vi "svfa_Tone Estimation (complex).vi"(8 "FFT size":i32, 9 "window size":i32, 10 "window":T1(ring), 11 "three fingers":cluster{"f0":dbl, "df":dbl, "spectrum":cdb[]}={"f0"=0.0, "df"=1.0, "spectrum"=[]} {"spectrum" format="%.2f"; "df" format="%.2f"; "f0" format="%.5f"}) -> (3 "single tone info.":T2 {"phase [degree]" format="%.2f"; "amplitude" format="%_6f"; "frequency" format="%_16e"})   [LabVIEW 2017]
doc: "This VI takes the three domainent FFT bins to apply the Newton-Raphson's root finding algorithm to determine the exact frequency, phase and amplitude.\nThe input is not necessary \"three fingers\", it could be two, four, or more."
uses:
  <vilib>/addons/_NISVFA/_Spectrum Processing/subVIs/svfa_Tone Estimation Subroutine G(f) (complex).vi
  <vilib>/addons/_NISVFA/_Spectrum Processing/subVIs/svfa_Window Frequency Response.vi
  <vilib>/addons/_NISVFA/_Spectrum Processing/subVIs/svfa_Window Frequency Response (double array).vi
  <vilib>/Analysis/baseanly.llb/Dot Product.vi
  <vilib>/Analysis/baseanly.llb/Complex Dot Product.vi
  <vilib>/addons/_NISVFA/_Spectrum Processing/subVIs/svfa_Rect Window Frequency Response.vi
  <vilib>/addons/_NISVFA/_Spectrum Processing/subVIs/svfa_Tone Estimation Subroutine G(f) (first derivative) (complex).vi
  <vilib>/addons/_NISVFA/_Spectrum Processing/subVIs/svfa_Cosine Window Coefficients.vi
  <vilib>/addons/_NISVFA/_Spectrum Processing/subVIs/svfa_Initial Guess for Tone Estimation (complex).vi
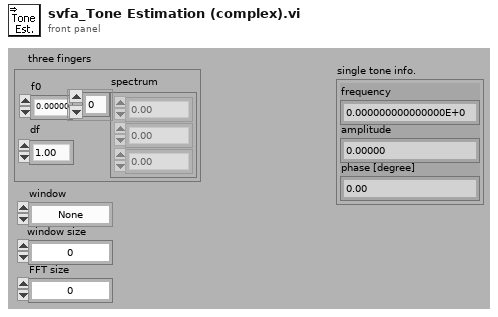
[diagram p1: front panel]
types:
  T1 = enum16{"None ", "Hanning", "Hamming", "Blackman-Harris", "Exact Blackman", "Blackman", "Flat Top", "4 Term B-Harris ", "7 Term B-Harris", "Low Sidelobe"}
  T2 = cluster{"frequency":dbl, "amplitude":dbl, "phase [degree]":dbl}
  T3 = cluster{"initial guess":dbl, "Amplitude":dbl, "initial guess":dbl}
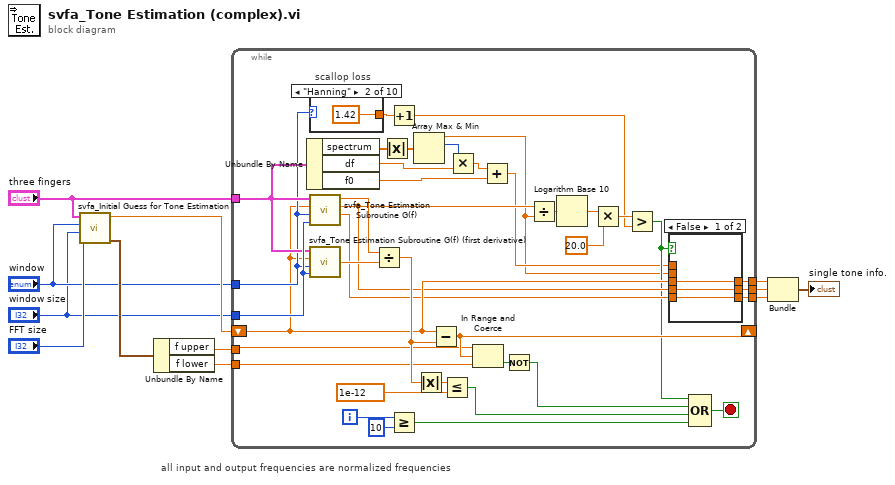
[diagram p0: block diagram]
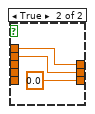
[diagram p2: hidden frame]
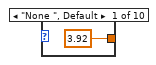
[diagram p3: hidden frame]
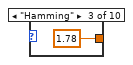
[diagram p4: hidden frame]
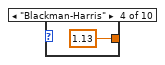
[diagram p5: hidden frame]
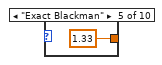
[diagram p6: hidden frame]
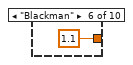
[diagram p7: hidden frame]
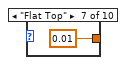
[diagram p8: hidden frame]
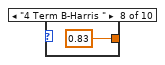
[diagram p9: hidden frame]
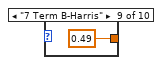
[diagram p10: hidden frame]
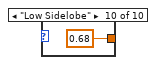
[diagram p11: hidden frame]
diagram:
  # "all input and output frequencies are normalized frequencies"
  n1 = call-poly <vilib>:"svfa_Initial Guess for Tone Estimation.vi"("FFT size"="FFT size", "window size"="window size", "window"="window", "three fingers"="three fingers") -> ("range"=w5:cluster{"f upper":dbl, "f lower":dbl}, "initial guess"=w4:dbl)  [unwired: 6 in]
  n2 = Unbundle By Name(w5) -> ("f upper"=w9:dbl, "f lower"=w8:dbl)
  n3 = while {
    tunnel: "three fingers" -> [w36]
    tunnel: w8 -> [w38]
    tunnel: "window size" -> [w37]
    tunnel: "window" -> [w33]
    tunnel: w9 -> [w39]
    tunnel: [w25] -> w11
    tunnel: [w26] -> w10
    tunnel: [w27] -> w7
    shift-left: w4 -> [w30]
    shift-right: [w41] -> _
    i -> [w45]
    stop <- w47 stop-if-true
    # "scallop loss"
    n4 = Unbundle By Name(w36) -> ("spectrum"=w35:cdb[], "df"=w21:dbl, "f0"=w20:dbl)
    n5 = case shown="\"Hanning\"" w33 {
      tunnel: [3.92 ("y") 1.42 ("y") 1.78 ("y") 1.13 ("y") 1.33 ("y") 1.1 ("y") 0.01 ("y") 0.83 ("y") 0.49 ("y") 0.68 ("y")] -> w31
      frame "None ", Default {
      }
      frame "Hanning" {
      }
      frame "Hamming" {
      }
      frame "Blackman-Harris" {
      }
      frame "Exact Blackman" {
      }
      frame "Blackman" {
      }
      frame "Flat Top" {
      }
      frame "4 Term B-Harris " {
      }
      frame "7 Term B-Harris" {
      }
      frame "Low Sidelobe" {
      }
    }
    n6 = call-poly <vilib>:"svfa_Tone Estimation Subroutine G(f).vi"("N (window length)"=w37, "window"=w33, "frequency"=w30, "three fingers"=w36) -> ("phase [degree]"=w28:dbl, "Amplitude"=w29:dbl, "G(f)"=w42:dbl)  [unwired: 1 in]
    n7 = call-poly <vilib>:"svfa_Tone Estimation Subroutine G(f) (first derivative).vi"("N (window length)"=w37, "window"=w33, "frequency"=w30, "three fingers"=w36) -> ("G'(f)"=w51:dbl)
    n8 = Divide(x=w42, y=w51) -> (x/y=w46:dbl)
    n9 = Absolute Value(x=w35) -> (abs(x)=w34:dbl[])
    n10 = Increment(x=w31) -> (x+1=w13:dbl)
    n11 = Greater Or Equal?(x=w45, y=10) -> (x >= y?=w48:bool)
    n12 = Array Max & Min(array=w34) -> (max value=w17:dbl, max index (indices)=w22:i32)  [unwired: 2 out]
    n13 = Absolute Value(x=w46) -> (abs(x)=w49:dbl)
    n14 = Subtract(x=w30, y=w46) -> (x-y=w41:dbl)
    n15 = Less Or Equal?(x=w49, y=1e-12) -> (x <= y?=w43:bool)
    n16 = Multiply(x=w22, y=w21) -> (x*y=w19:dbl)
    n17 = In Range and Coerce(upper limit=w39, x=w41, lower limit=w38) -> (In Range?=w40:bool)  [unwired: 1 out]
    n18 = Add(x=w19, y=w20) -> (x+y=w18:dbl)
    n19 = Not(x=w40) -> (.not. x?=w24:bool)
    n20 = Divide(x=w29, y=w17) -> (x/y=w32:dbl)
    n21 = Logarithm Base 10(1:w32) -> (0:w16:dbl)
    n22 = Multiply(x=w16, y=20.0) -> (x*y=w15:dbl)
    n23 = Greater?(x=w15, y=w13) -> (0:w23:bool)
    n24 = case shown="False" w23 {
      tunnel: w30 -> [w54 _]
      tunnel: w29 -> [w53 _]
      tunnel: w28 -> [w52 _]
      tunnel: [w54 w56] -> w27
      tunnel: [w53 w55] -> w26
      tunnel: [w52 0.0 ("initial guess")] -> w25
      tunnel: w18 -> [_ w56]
      tunnel: w17 -> [_ w55]
      frame False {
      }
      frame True {
      }
    }
    n25 = Compound Arithmetic op=OR(w23, w24, w43, w48) -> (w47:bool)
  }
  n26 = Bundle("initial guess"=w7, "Amplitude"=w10, "initial guess"=w11) -> (→"single tone info.":T3)  [unwired: 1 in]
